vi "ESPECTROSCOPIA.vi"() -> ()   [LabVIEW 2016]
uses:
  Control 1.ctl
  <vilib>/userdefined/High Color/IMAQdx.ctl
  <vilib>/vision/driver/NI_Vision_Acquisition_Software.lvlib
panel:
  in  "worksheet index (0)":i32
  in  "entrada de datos desde un archivo":bool
  in  "Observar cámara":bool
  in  "Control de espejos":T1={"Movimiento de spot en y"=0.78, "Movimiento de spot en x"=0.5255, "tipo "=enum."barrido", "yFin"=0.82, "Paso"=0.01, "xFin"=0.5655} {"Movimiento de spot en x" scale=-10.0..10.0; "Movimiento de spot en y" min=-10.0 max=10.0 scale=-10.0..10.0}
  in  "arreglo opciones":bool[](array[boolean])=[FALSE, TRUE, TRUE, TRUE, FALSE]
  in  "Control CCD":T2={"Numero de lecturas"=0, "tiempo de lectura (ms)"=100, "Exposure"=0.053229, "Valor Gamma"=1.0, "Ganancia"=33, "Opción"=enum."Espectro", "VISA resource name"="", "Enable Strobe (Disabled)"=FALSE} {"Ganancia" min=0 max=100; "Valor Gamma" min=1.0 max=2.2; "Exposure" min=5e-05 max=0.053229}
  in  "Guardar":bool=TRUE
  in  "valor delay":u32=300
  in  "tiempo de avance":u32=300
  in  "Orden":T3(array[ring])=[enum."espejos", enum."voltaje", enum."polarizador", enum."CCD"]
  in  "Nombre del archivo":string="prueba280519PASO0.01_01_03"
  in  "stop medición":bool
  in  "stop":bool
  in  "Iniciar medición":bool
  in  "Config. fotodiodo y potenciometro":T4={"tiempo. lect."=300, "num. med"=20, "tiempo. lectura"=0, "average rate"=0, "Readout Config"="POW", "Tipo de Medición"=enum."Lockin", "usar multimetro"=FALSE}
  in  "config. Polarizador":T5={"pos inic"=0.0, "pos.final"=5.0, "incremento"=1.0, "velocidad"=0.0}
  in  "Config. voltaje y corriente":T6 {"Measurement Function (0:Voltage)" items=["Voltage", "Current", "Power"]; "Unit(V)" items=["V", "mV", "kV", "A", "mA"]; "Function(0:Voltage)" items=["Voltage", "Current"]}
  out "Imagen":T7(plugin-control)
  out "MULTÍMETRO":dbl format="%^#_9e"
  out "valor potenciometro":dbl format="%^#_9e"
  out "LockIn":dbl
  out "Valor voltaje":dbl
  out "corriente":dbl
  out "Ángulo del polarizador":dbl
  out "ysal":dbl=0.78
  out "xsal":dbl=0.5255
  out "division":T8
  out "multímetro":T8
  in  "Gráficas visibles":bool[](array[boolean])=[TRUE, FALSE, FALSE, FALSE, FALSE]
  in  "SerialNumber":string="55000538"
  out "I-V":cluster{dbl[], dbl[]}(graph)
  out "Gráfica general":T8
  out "Power meter":cluster{dbl[], dbl[]}(graph)
  # "Espejos"
  # "Polarizador"
  # "Fuente voltaje"
  # "Lockin \npotenciometro"
  # "CCD"
  # "Espectro"
  # "Imágen"
  # "Amplificador Lock in"
  # "potenciometro"
  # "Valores Numéricos"
  # "Gráfica general"
  # "Gráfica potenciómetro"
  # "Gráfica I-V"
  # "Multimetro"
  # "lockin/multimetro"
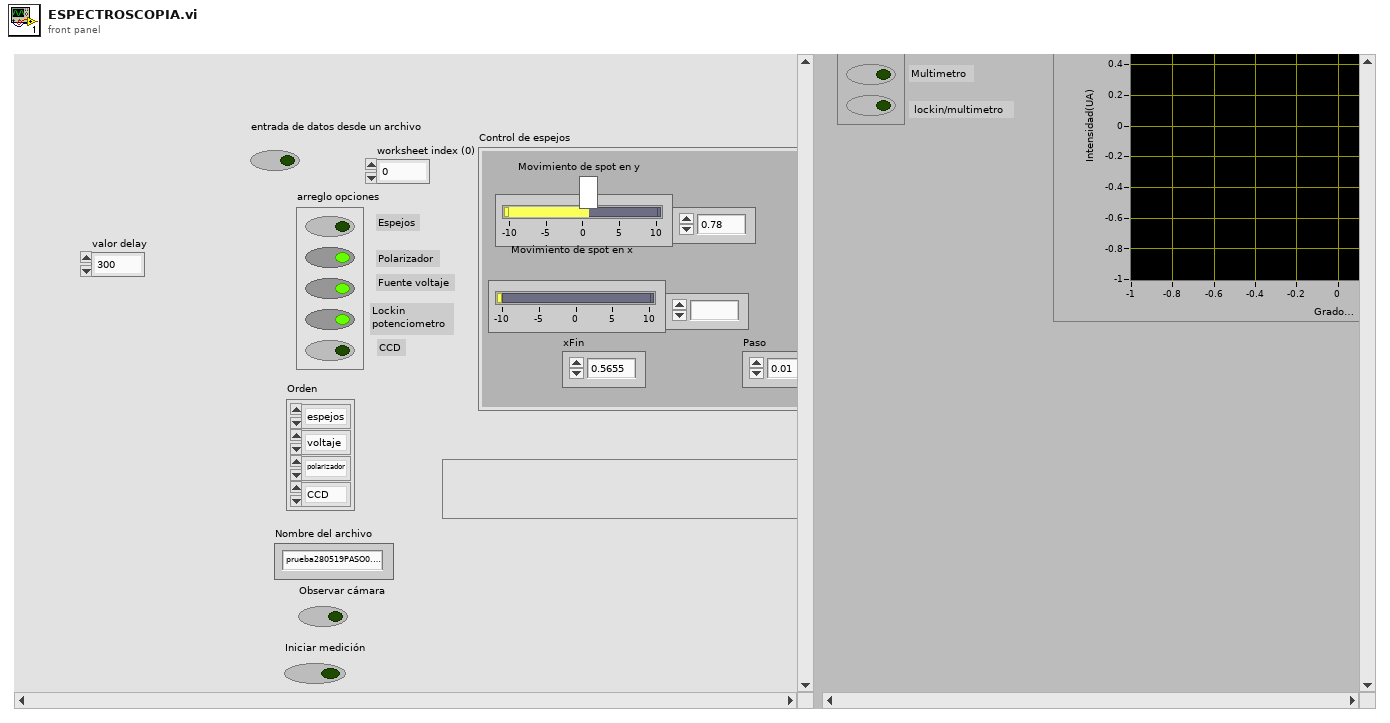
[diagram p1: front panel]
types:
  T1 = cluster{"Movimiento de spot en y":dbl, "Movimiento de spot en x":ext, "tipo ":enum16{"manual", "barrido"}, "yFin":dbl, "Paso":dbl, "xFin":dbl}
  T2 = cluster{"Numero de lecturas":i32, "tiempo de lectura (ms)":u32, "Exposure":dbl, "Valor Gamma":dbl, "Ganancia":i64, "Opción":enum16{"Espectro", "Imágen"}, "VISA resource name":refnum<visa-resource-name>, "Enable Strobe (Disabled)":bool}
  T3 = enum16{"espejos", "polarizador", "voltaje", "potenciometro y lockin", "CCD"}[]
  T4 = cluster{"tiempo. lect.":i32, "num. med":i32, "tiempo. lectura":i32, "average rate":i32, "Readout Config":string, "Tipo de Medición":enum16{"Lockin", "Lockin-potenciometro", "Potenciometro"}, "usar multimetro":bool}
  T5 = cluster{"pos inic":dbl, "pos.final":dbl, "incremento":dbl, "velocidad":dbl}
  T6 = cluster{"Voltaje inicial":dbl, "incremento":dbl, " voltaje final":dbl, "Function(0:Voltage)":u16, "Unit(V)":u16, "Measurement Function (0:Voltage)":u16, "VISA resource name":refnum<visa-resource-name>}
  T7 = typedef "IMAQ Image.ctl" = refnum<image>
  T8 = typedef "Control 1.ctl" = cluster{dbl[], dbl[]}
  T9 = typedef "IMAQdx.ctl" = refnum<k21>
  T10 = enum16{"espejos", "polarizador", "voltaje", "potenciometro y lockin", "CCD"}
  T11 = enum16{"Lockin", "Lockin-potenciometro", "Potenciometro"}
  T12 = cluster{"Global Rectangle":i32[], "Contours":cluster{"Contour Type":u32, "ROI Type":u32, "Points":i32[]}[]}
  T13 = cluster{"Wavelength (nm)":dbl[], "arreglo promedio":dbl[]}
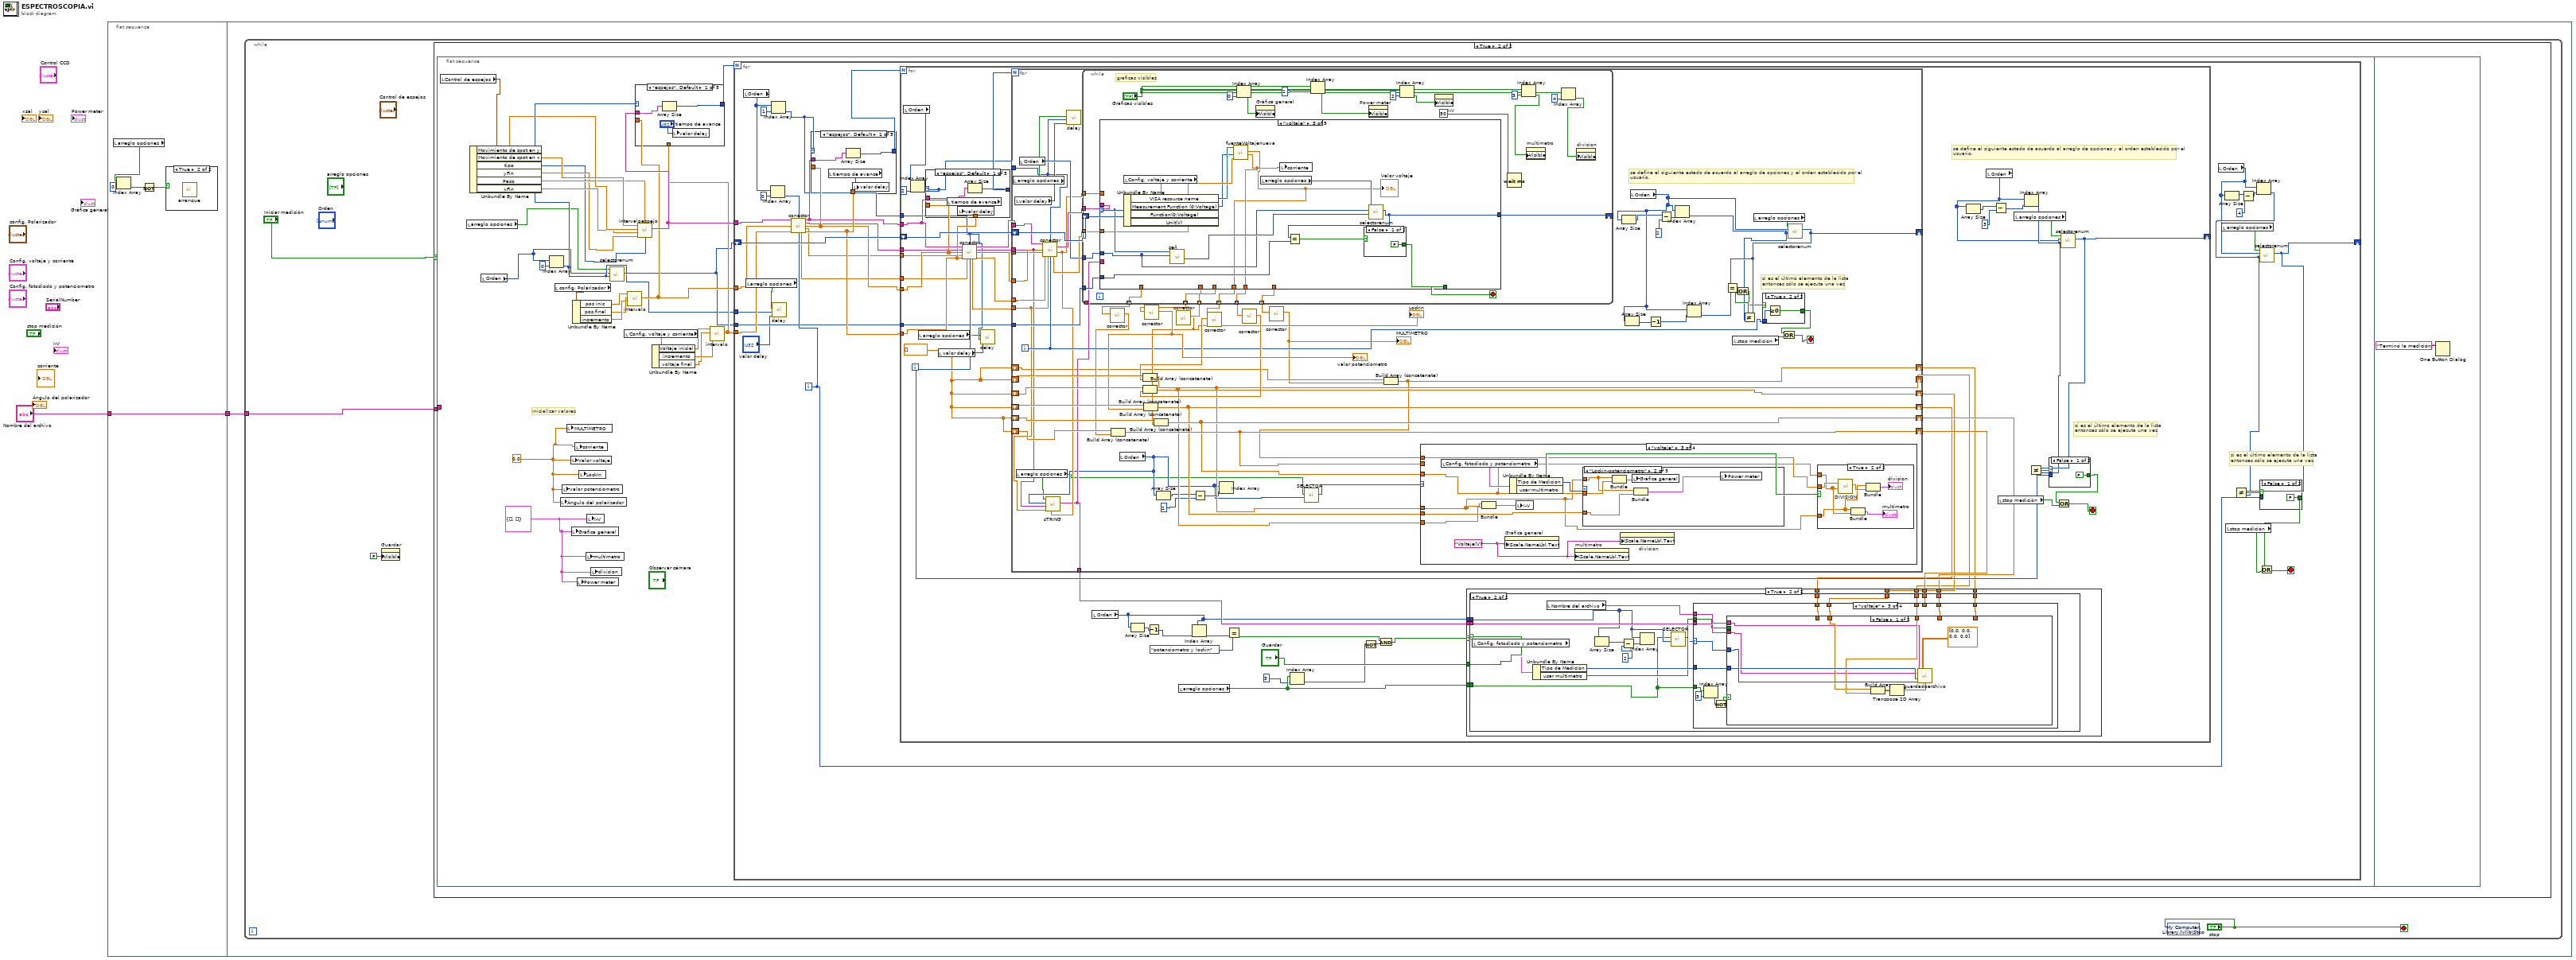
[diagram p0: block diagram]
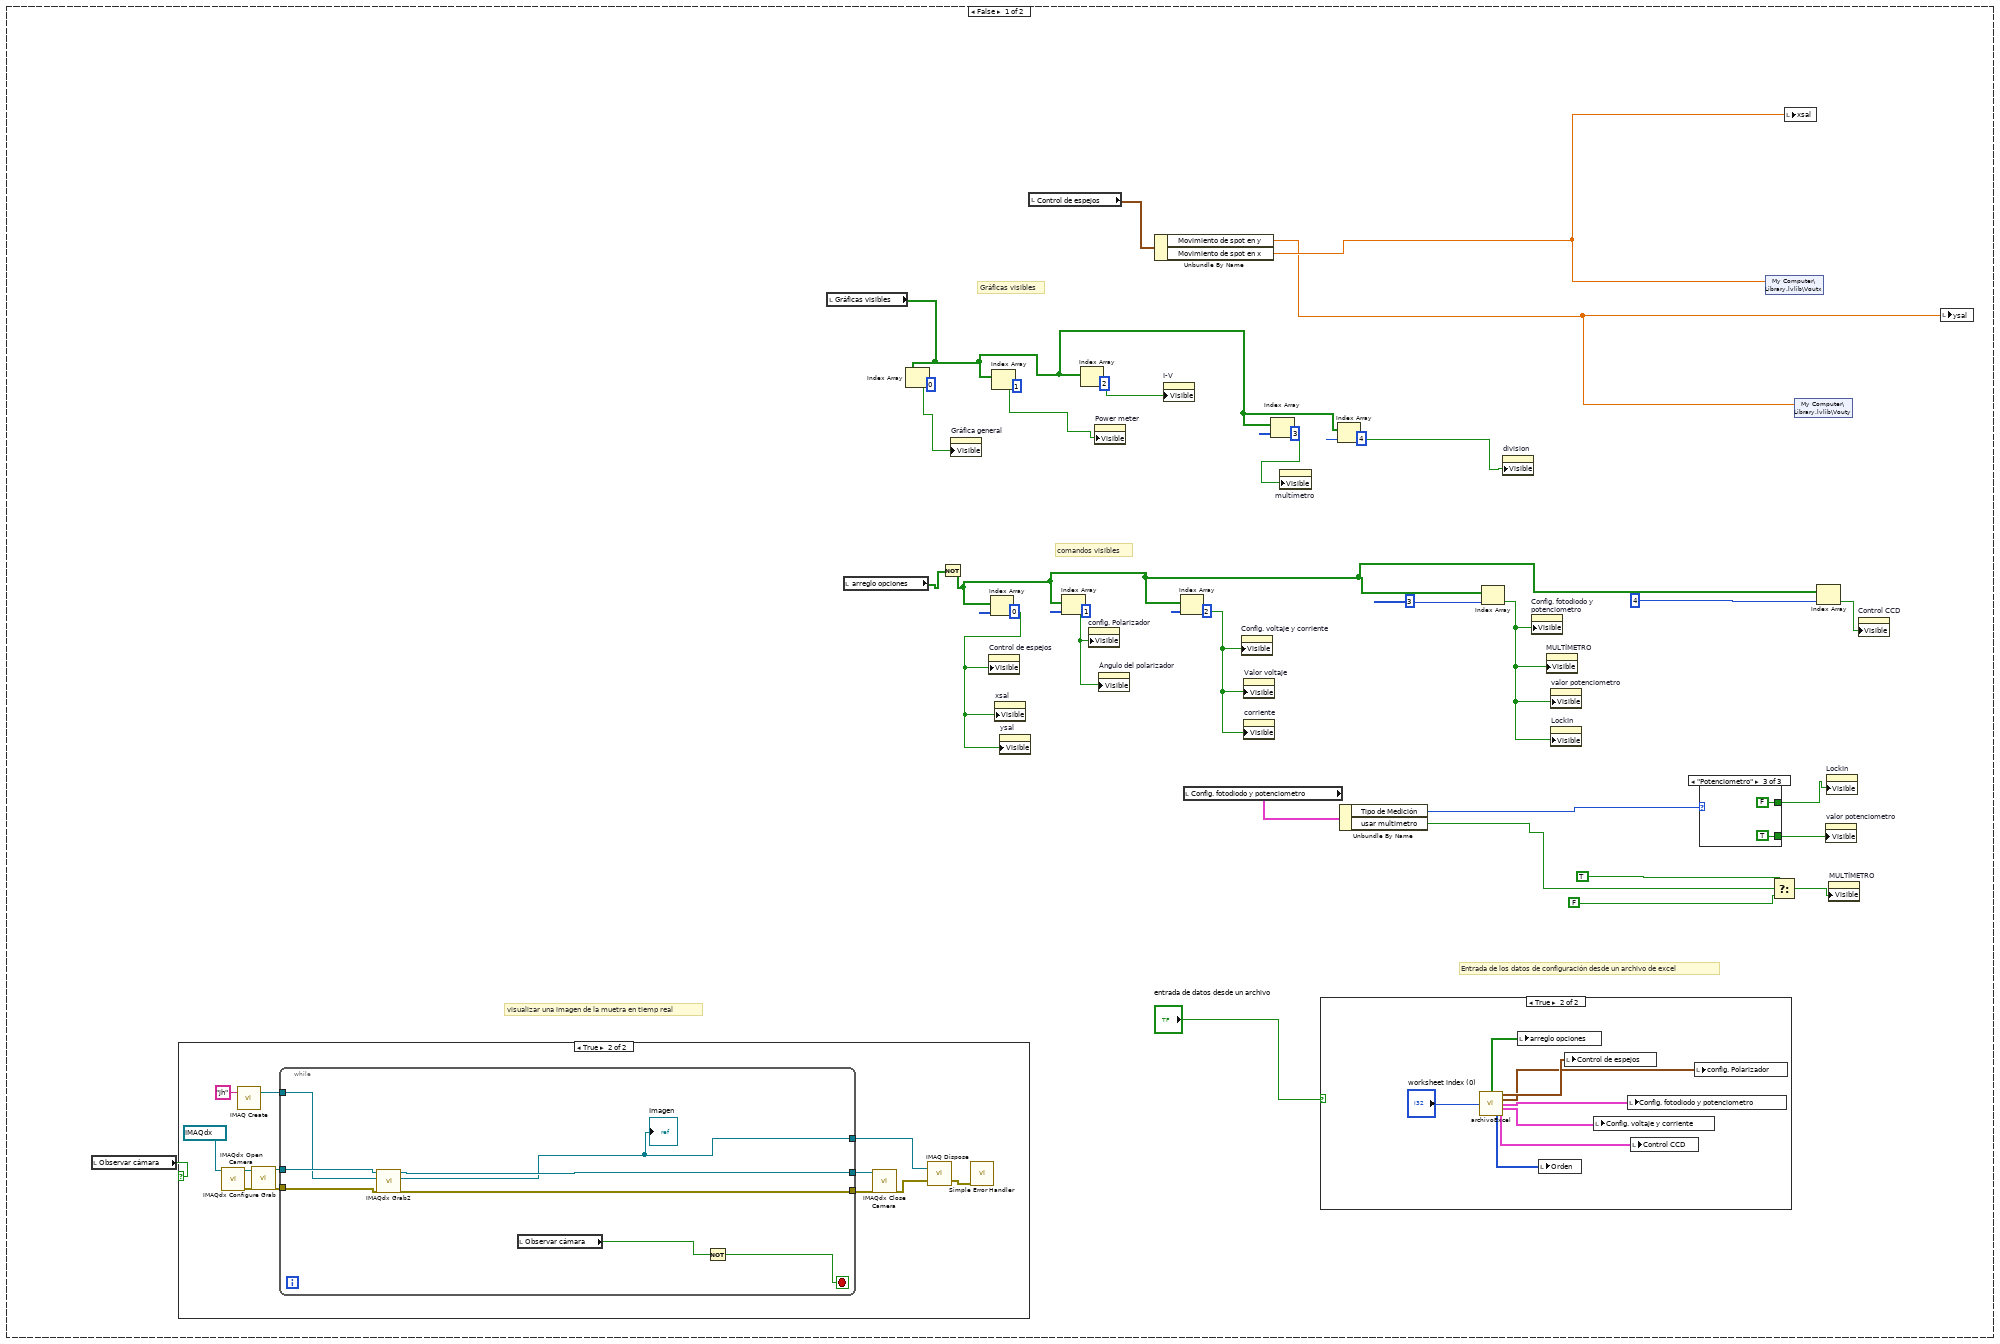
[diagram p3: hidden frame]
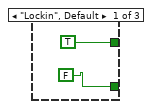
[diagram p6: hidden frame]
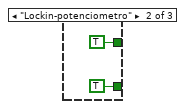
[diagram p7: hidden frame]
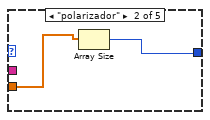
[diagram p8: hidden frame]
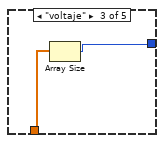
[diagram p9: hidden frame]
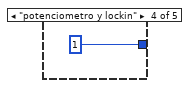
[diagram p10: hidden frame]
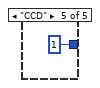
[diagram p11: hidden frame]
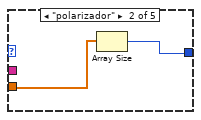
[diagram p12: hidden frame]
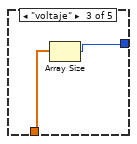
[diagram p13: hidden frame]
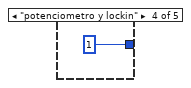
[diagram p14: hidden frame]
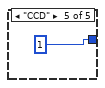
[diagram p15: hidden frame]
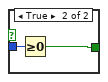
[diagram p16: hidden frame]
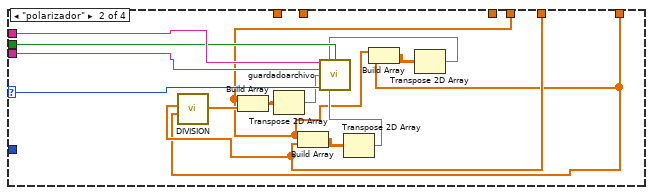
[diagram p20: hidden frame]
diagram:
  n1 = flat-sequence {
    tunnel: "Nombre del archivo" -> [w7]
    tunnel: [w7] -> w1
    tunnel: w1 -> [w8]
    frame #0 {
      n2 = local read "arreglo opciones"() -> (w6:bool[])
      n3 = Index Array(array=w6, index=0) -> (element=w3:bool)
      n4 = Not(x=w3) -> (.not. x?=w4:bool)
      n5 = case shown="True" w4 {
        frame False {
        }
        frame True {
          n6 = call "arranque.vi"() -> ()  [unwired: 12 in]
        }
      }
    }
    frame #1 {
      n7 = while {
        tunnel: w8 -> [w10]
        stop <- "stop" stop-if-true
        n8 = property on="Guardar" class="Bool (strict)"("Visible"=FALSE) -> ()  [unwired: 2 in, 2 out]
        n9 = case shown="True" "Iniciar medición" {
          tunnel: w10 -> [_ w83]
          frame False {
            # "Entrada de los datos de configuración desde un archivo de excel"
            # "visualizar una imagen de la muetra en tiemp real"
            # "comandos visibles"
            # "Gráficas visibles"
            n10 = local read "Observar cámara"() -> (w15:bool)
            n11 = case shown="True" w15 {
              frame False {
              }
              frame True {
                n12 = call <vilib>:"IMAQdx Open Camera.vi"("Session In"=T9 "cam4") -> ("error out"=w68:errorcluster, "Session Out"=w67:T9)  [unwired: 9 in]
                n13 = call "IMAQ Create"("Image Name"="jh") -> ("New Image"=w63:T7)  [unwired: 4 in, 1 out]
                n14 = call <vilib>:"IMAQdx Configure Grab.vi"("error in"=w68, "Session In"=w67) -> ("error out"=w65:errorcluster, "Session Out"=w66:T9)  [unwired: 8 in]
                n15 = while {
                  tunnel: w66 -> [w76]
                  tunnel: w65 -> [w75]
                  tunnel: w63 -> [w74]
                  tunnel: [w73] -> w61
                  tunnel: [w72] -> w60
                  tunnel: [w69] -> w58
                  stop <- w70 stop-if-true
                  n16 = call <vilib>:"IMAQdx Grab2.vi"("error in"=w75, "Image In"=w74, "Session In"=w76) -> ("error out"=w72:errorcluster, "Image Out"=w69:T7, "Session Out"=w73:T9)  [unwired: 5 in, 1 out]
                  "Imagen" <- w69
                  n17 = local read "Observar cámara"() -> (w71:bool)
                  n18 = Not(x=w71) -> (.not. x?=w70:bool)
                }
                n19 = call <vilib>:"IMAQdx Close Camera.vi"("error in"=w60, "Session In"=w61) -> ("error out"=w59:errorcluster)  [unwired: 9 in]
                n20 = call "IMAQ Dispose"("Image"=w58, "error in (no error)"=w59) -> ("error out"=w57:errorcluster)  [unwired: 4 in]
                n21 = call <vilib>:"Simple Error Handler.vi"("error in (no error)"=w57) -> ()  [unwired: 4 in, 5 out]
              }
            }
            n22 = local read "Gráficas visibles"() -> (w40:bool[])
            n23 = local read "arreglo opciones"() -> (w17:bool[])
            n24 = Index Array(array=w40, index=0) -> (element=w45:bool)
            n25 = Not(x=w17) -> (.not. x?=w16:bool[])
            n26 = property on="Gráfica general" class="XYGraph (strict)"("Visible"=w45) -> ()  [unwired: 2 in, 2 out]
            n27 = Index Array(array=w16, index=0) -> (element=w14:bool)
            n28 = property on="Control de espejos" class="Clust (strict)"("Visible"=w14) -> ()  [unwired: 2 in, 2 out]
            n29 = Index Array(array=w40, index=1) -> (element=w44:bool)
            n30 = property on="xsal" class="DigNum (strict)"("Visible"=w14) -> ()  [unwired: 2 in, 2 out]
            n31 = property on="ysal" class="DigNum (strict)"("Visible"=w14) -> ()  [unwired: 2 in, 2 out]
            n32 = local read "Control de espejos"() -> (w20:T1)
            n33 = Index Array(array=w16, index=1) -> (element=w35:bool)
            n34 = Index Array(array=w40, index=2) -> (element=w43:bool)
            n35 = property on="config. Polarizador" class="Clust (strict)"("Visible"=w35) -> ()  [unwired: 2 in, 2 out]
            n36 = property on="Power meter" class="XYGraph (strict)"("Visible"=w44) -> ()  [unwired: 2 in, 2 out]
            n37 = property on="Ángulo del polarizador" class="DigNum (strict)"("Visible"=w35) -> ()  [unwired: 2 in, 2 out]
            n38 = Unbundle By Name(w20) -> ("Movimiento de spot en y"=w18:dbl, "Movimiento de spot en x"=w19:ext)
            n39 = property on="I-V" class="XYGraph (strict)"("Visible"=w43) -> ()  [unwired: 2 in, 2 out]
            n40 = Index Array(array=w16, index=2) -> (element=w33:bool)
            n41 = local read "Config. fotodiodo y potenciometro"() -> (w28:T4)
            n42 = property on="Config. voltaje y corriente" class="Clust (strict)"("Visible"=w33) -> ()  [unwired: 2 in, 2 out]
            n43 = property on="Valor voltaje" class="DigNum (strict)"("Visible"=w33) -> ()  [unwired: 2 in, 2 out]
            n44 = property on="corriente" class="DigNum (strict)"("Visible"=w33) -> ()  [unwired: 2 in, 2 out]
            n45 = Index Array(array=w40, index=3) -> (element=w38:bool)
            n46 = property on="multímetro" class="XYGraph (strict)"("Visible"=w38) -> ()  [unwired: 2 in, 2 out]
            n47 = case shown="True" "entrada de datos desde un archivo" {
              frame False {
              }
              frame True {
                n48 = call "archivoExcel.vi"("worksheet index (0)"="worksheet index (0)") -> ("opciones"=w56:bool[], "Control de espejos 3"=w55:T1, "config. Polarizador 2"=w54:T5, "Config. fotodiodo y potenciometro 2"=w53:T4, "Config. voltaje y corriente 2"=w52:T6, "orden 2"=w50:T3, "Control CCD 2"=w51:T2)  [unwired: 8 in]
                n49 = local write "arreglo opciones"(w56) -> ()
                n50 = local write "Orden"(w50) -> ()
                n51 = local write "Control de espejos"(w55) -> ()
                n52 = local write "Config. voltaje y corriente"(w52) -> ()
                n53 = local write "Config. fotodiodo y potenciometro"(w53) -> ()
                n54 = local write "Control CCD"(w51) -> ()
                n55 = local write "config. Polarizador"(w54) -> ()
              }
            }
            n56 = Index Array(array=w40, index=4) -> (element=w39:bool)
            n57 = Unbundle By Name(w28) -> ("Tipo de Medición"=w27:T11, "usar multimetro"=w23:bool)
            n58 = Index Array(array=w16, index=3) -> (element=w31:bool)
            n59 = property on="division" class="XYGraph (strict)"("Visible"=w39) -> ()  [unwired: 2 in, 2 out]
            n60 = property on="Config. fotodiodo y potenciometro" class="Clust (strict)"("Visible"=w31) -> ()  [unwired: 2 in, 2 out]
            n61 = property on="MULTÍMETRO" class="DigNum (strict)"("Visible"=w31) -> ()  [unwired: 2 in, 2 out]
            n62 = property on="valor potenciometro" class="DigNum (strict)"("Visible"=w31) -> ()  [unwired: 2 in, 2 out]
            n63 = property on="LockIn" class="DigNum (strict)"("Visible"=w31) -> ()  [unwired: 2 in, 2 out]
            n64 = case shown="\"Potenciometro\"" w27 {
              tunnel: [TRUE TRUE FALSE] -> w26
              tunnel: [FALSE TRUE TRUE] -> w25
              frame "Lockin", Default {
              }
              frame "Lockin-potenciometro" {
              }
              frame "Potenciometro" {
              }
            }
            n65 = shared-variable "My Computer\\Library.lvlib\\Voutx"(w19) -> ()  [unwired: 1 in, 1 out]
            n66 = Select(t=TRUE, s=w23, f=FALSE) -> (s? t:f=w24:bool)
            n67 = local write "xsal"(w19) -> ()
            n68 = shared-variable "My Computer\\Library.lvlib\\Vouty"(w18) -> ()  [unwired: 1 in, 1 out]
            n69 = Index Array(array=w16, index=4) -> (element=w29:bool)
            n70 = property on="valor potenciometro" class="DigNum (strict)"("Visible"=w25) -> ()  [unwired: 2 in, 2 out]
            n71 = property on="LockIn" class="DigNum (strict)"("Visible"=w26) -> ()  [unwired: 2 in, 2 out]
            n72 = property on="MULTÍMETRO" class="DigNum (strict)"("Visible"=w24) -> ()  [unwired: 2 in, 2 out]
            n73 = property on="Control CCD" class="Clust (strict)"("Visible"=w29) -> ()  [unwired: 2 in, 2 out]
            n74 = local write "ysal"(w18) -> ()
          }
          frame True {
            n75 = flat-sequence {
              tunnel: w83 -> [_]
              frame #0 {
                w87 = cluster{dbl[], dbl[]} {[], []} ("I-V")
                w94 = 0.0
                # "Inicializar valores"
                n76 = local read "Control de espejos"() -> (w86:T1)
                n77 = local read "arreglo opciones"() -> (w85:bool[])
                n78 = Unbundle By Name(w86) -> ("Movimiento de spot en y"=w92:dbl, "Movimiento de spot en x"=w93:ext, "tipo"=w88:enum16{"manual", "barrido"}, "yFin"=w89:dbl, "Paso"=w91:dbl, "xFin"=w90:dbl)
                n79 = local read "Orden"() -> (w84:T3)
                n80 = Index Array(array=w84, index=0) -> (element=w95:T10)
                n81 = local read "config. Polarizador"() -> (w109:T5)
                n82 = local write "Ángulo del polarizador"(w94) -> ()
                n83 = local write "valor potenciometro"(w94) -> ()
                n84 = local write "MULTÍMETRO"(w94) -> ()
                n85 = local write "Valor voltaje"(w94) -> ()
                n86 = local write "Gráfica general"(w87) -> ()
                n87 = Unbundle By Name(w109) -> ("pos inic"=w108:dbl, "pos.final"=w106:dbl, "incremento"=w107:dbl)
                n88 = local write "corriente"(w94) -> ()
                n89 = local write "Power meter"(w87) -> ()
                n90 = local write "LockIn"(w94) -> ()
                n91 = local write "multímetro"(w87) -> ()
                n92 = local write "I-V"(w87) -> ()
                n93 = local write "division"(w87) -> ()
                n94 = call "selectorenum.vi"("Enum entrada"=w95, "Orden"=w84, "arreglo opciones"=w85) -> ("enum salida"=w96:T10)  [unwired: 8 in]
                n95 = local read "Config. voltaje y corriente"() -> (w105:T6)
                n96 = call "intervalo.vi"("incremento"=w107, "fin"=w106, "inicio"=w108) -> ("Array"=w98:dbl[])  [unwired: 8 in]
                n97 = call "intervaloespejo.vi"("tipo"=w88, "intervalo"=w91, "fin y"=w89, "fin x"=w90, "inicio y"=w92, "inicio x"=w93) -> ("salida"=w99:string[])  [unwired: 5 in]
                n98 = Unbundle By Name(w105) -> ("Voltaje inicial"=w104:dbl, "incremento"=w103:dbl, "voltaje final"=w102:dbl)
                n99 = call "intervalo.vi"("incremento"=w103, "fin"=w102, "inicio"=w104) -> ("Array"=w97:dbl[])  [unwired: 8 in]
                n100 = case shown="\"espejos\", Default" w95 {
                  tunnel: [w111 w113 w115 1 1] -> w100
                  tunnel: w99 -> [w112 _ _ _ _]
                  tunnel: w98 -> [_ w114 _ _ _]
                  tunnel: w97 -> [_ _ w116 _ _]
                  frame "espejos", Default {
                    n101 = Array Size(array=w112) -> (size(s)=w111:i32)
                    n102 = local write "valor delay"("tiempo de avance") -> ()
                  }
                  frame "polarizador" {
                    n103 = Array Size(array=w114) -> (size(s)=w113:i32)
                  }
                  frame "voltaje" {
                    n104 = Array Size(array=w116) -> (size(s)=w115:i32)
                  }
                  frame "potenciometro y lockin" {
                  }
                  frame "CCD" {
                  }
                }
                n105 = for {
                  N: w100 -> [_]
                  tunnel: w99 -> [w140]
                  shift-right: [w147] -> _
                  shift-left: w96 -> [w150]
                  tunnel: w98 -> [w139]
                  tunnel: w97 -> [w138]
                  tunnel: w96 -> [w130]
                  tunnel: w95 -> [w126]
                  i -> [w137]
                  stop <- w144 stop-if-true
                  # "si es el último elemento de la lista\nentonces sólo se ejecuta una vez"
                  n106 = local read "Orden"() -> (w129:T3)
                  n107 = local read "arreglo opciones"() -> (w125:bool[])
                  n108 = Index Array(array=w129, index=0) -> (element=w119:T10)
                  n109 = Index Array(array=w129, index=1) -> (element=w127:T10)
                  n110 = call "delay.vi"("valor delay"="valor delay", "element"=w126, "arreglo opciones"=w125) -> ()  [unwired: 9 in]
                  n111 = call "conector.vi"("salida"=w140, "Enum 2"=w119, "polarizador"=w139, "voltaje"=w138, "Indice"=w137) -> ("salida 2"=w136:string[], "Salida ent 2"=w133:string, "polarizador 2"=w135:dbl[], "Polarizador"=w132:dbl, "VoltajeEnt 2"=w131:dbl, "voltaje 2"=w134:dbl[])  [unwired: 5 in]
                  n112 = case shown="\"espejos\", Default" w127 {
                    tunnel: [w152 w154 w156 1 1] -> w143
                    tunnel: w136 -> [w153 _ _ _ _]
                    tunnel: w135 -> [_ w155 _ _ _]
                    tunnel: w134 -> [_ _ w157 _ _]
                    frame "espejos", Default {
                      n113 = local read "tiempo de avance"() -> (w151:u32)
                      n114 = Array Size(array=w153) -> (size(s)=w152:i32)
                      n115 = local write "valor delay"(w151) -> ()
                    }
                    frame "polarizador" {
                      n116 = Array Size(array=w155) -> (size(s)=w154:i32)
                    }
                    frame "voltaje" {
                      n117 = Array Size(array=w157) -> (size(s)=w156:i32)
                    }
                    frame "potenciometro y lockin" {
                    }
                    frame "CCD" {
                    }
                  }
                  n118 = for {
                    N: w143 -> [_]
                    tunnel: w136 -> [w201]
                    shift-right: [w213] -> _
                    shift-left: w150 -> [w215]
                    tunnel: w135 -> [w200]
                    tunnel: w134 -> [w199]
                    tunnel: w133 -> [w197]
                    tunnel: w132 -> [w196]
                    tunnel: w131 -> [w195]
                    tunnel: w130 -> [w194]
                    tunnel: w127 -> [w163]
                    i -> [w198]
                    stop <- w212 stop-if-true
                    w174 = dbl[] []
                    # "si es el último elemento de la lista\nentonces sólo se ejecuta una vez"
                    # "se define el siguiente estado de acuerdo al arreglo de opciones y el orden establecido por el \nusuario."
                    n119 = local read "Orden"() -> (w207:T3)
                    n120 = Index Array(array=w207, index=2) -> (element=w193:T10)
                    n121 = local read "arreglo opciones"() -> (w192:bool[])
                    n122 = case shown="\"espejos\", Default" w193 {
                      tunnel: [w302 w304 w306 1 1] -> w208
                      tunnel: w201 -> [w303 _ _ _ _]
                      tunnel: w200 -> [_ w305 _ _ _]
                      tunnel: w199 -> [_ _ w307 _ _]
                      frame "espejos", Default {
                        n123 = local read "tiempo de avance"() -> (w301:u32)
                        n124 = local write "valor delay"(w301) -> ()
                        n125 = Array Size(array=w303) -> (size(s)=w302:i32)
                      }
                      frame "polarizador" {
                        n126 = Array Size(array=w305) -> (size(s)=w304:i32)
                      }
                      frame "voltaje" {
                        n127 = Array Size(array=w307) -> (size(s)=w306:i32)
                      }
                      frame "potenciometro y lockin" {
                      }
                      frame "CCD" {
                      }
                    }
                    n128 = local read "valor delay"() -> (w191:u32)
                    n129 = call "conector.vi"("salida"=w201, "Enum 2"=w163, "Salida ent"=w197, "polarizador"=w200, "Polarizadorent"=w196, "voltaje"=w199, "VoltajeEnt"=w195, "Indice"=w198) -> ("salida 2"=w204:string[], "Salida ent 2"=w176:string, "polarizador 2"=w203:dbl[], "Polarizador"=w175:dbl, "VoltajeEnt 2"=w177:dbl, "voltaje 2"=w202:dbl[])  [unwired: 2 in]
                    n130 = call "delay.vi"("valor delay"=w191, "element"=w163, "arreglo opciones"=w192) -> ()  [unwired: 9 in]
                    n131 = for {
                      N: w208 -> [_]
                      shift-right: [w371] -> _
                      shift-left: w215 -> [w375]
                      tunnel: w204 -> [w352]
                      tunnel: w203 -> [w351]
                      tunnel: w202 -> [w350]
                      shift-right: [w338] -> w186
                      shift-left: w174 -> [w369]
                      shift-right: [w337] -> w187
                      shift-left: w174 -> [w368]
                      shift-right: [w336] -> w188
                      shift-left: w174 -> [w367]
                      shift-right: [w339] -> w189
                      shift-left: w174 -> [w366]
                      tunnel: w177 -> [w325]
                      tunnel: w175 -> [w346]
                      tunnel: w176 -> [w326]
                      tunnel: w194 -> [w344]
                      tunnel: w193 -> [w313]
                      shift-right: [w340] -> w190
                      shift-left: w174 -> [w342]
                      tunnel: [w322] -> w178
                      shift-right: [w319] -> w173
                      shift-left: w174 -> [w320]
                      i -> [w347]
                      stop <- w365 stop-if-true
                      # "si es el último elemento de la lista\nentonces sólo se ejecuta una vez"
                      # "se define el siguiente estado de acuerdo al arreglo de opciones y el orden establecido por el \nusuario."
                      n132 = local read "arreglo opciones"() -> (w334:bool[])
                      n133 = local read "valor delay"() -> (w333:u32)
                      n134 = local read "arreglo opciones"() -> (w314:bool[])
                      n135 = local read "Orden"() -> (w345:T3)
                      n136 = call "conector.vi"("salida"=w352, "Enum 2"=w313, "Salida ent"=w326, "polarizador"=w351, "Polarizadorent"=w346, "voltaje"=w350, "VoltajeEnt"=w325, "Indice"=w347) -> ("Salida ent 2"=w349:string, "Polarizador"=w324:dbl, "VoltajeEnt 2"=w348:dbl)  [unwired: 2 in, 3 out]
                      n137 = call "delay.vi"("valor delay"=w333, "element"=w313, "arreglo opciones"=w334) -> ()  [unwired: 9 in]
                      n138 = local read "Orden"() -> (w315:T3)
                      n139 = call "sTRING.vi"("angulo"=w324, "Valor del voltaje"=w325, "cadena entrada"=w326, "Orden"=w315, "arreglo opciones"=w314) -> ("String"=w322:string)  [unwired: 6 in]
                      n140 = while {
                        shift-right: [w444] -> _
                        shift-left: w375 -> [w445]
                        tunnel: w349 -> [w441]
                        tunnel: w324 -> [w442]
                        tunnel: w348 -> [w440]
                        tunnel: [w439] -> w359 mode=indexing
                        tunnel: [w438] -> w357 mode=indexing
                        tunnel: [w437] -> w360 mode=indexing
                        tunnel: [w436] -> w361 mode=indexing
                        tunnel: w345 -> [w434]
                        tunnel: w344 -> [w433]
                        tunnel: [w432] -> w343 mode=indexing
                        tunnel: w322 -> [w431]
                        tunnel: [w424] -> w321 mode=indexing
                        stop <- w443 stop-if-true
                        # "graficas visibles"
                        n141 = case shown="\"voltaje\"" w445 {
                          selector: w445 -> [w451 w462 w479 w492 w522]
                          tunnel: [w454 w466 w482 w504 w527] -> w444
                          tunnel: [w453 w468 w484 w505 w528] -> w443
                          tunnel: w442 -> [_ w465 _ _ _]
                          tunnel: w441 -> [w452 _ _ _ _]
                          tunnel: w440 -> [_ _ w474 _ _]
                          tunnel: [_ _ w475 _ _] -> w439
                          tunnel: [_ _ w476 _ _] -> w438
                          tunnel: [_ _ _ w502 _] -> w437
                          tunnel: [_ _ _ w501 _] -> w436
                          tunnel: w434 -> [w448 w461 w477 w490 w523]
                          tunnel: w433 -> [w449 w460 w480 w493 w526]
                          tunnel: [_ w459 _ _ _] -> w432
                          tunnel: w431 -> [_ _ _ _ w520]
                          tunnel: [_ _ _ w488 _] -> w424
                          frame "espejos", Default {
                            n142 = call "señ.vi"("Orden"=w448, "Enum"=w451) -> ("element"=w450:T10)  [unwired: 9 in]
                            n143 = call "controlespejo.vi"("cadena entrada"=w452) -> ("x"=w447:dbl, "y"=w446:dbl)  [unwired: 9 in]
                            n144 = local write "xsal"(w447) -> ()
                            n145 = local write "ysal"(w446) -> ()
                            n146 = local read "arreglo opciones"() -> (w456:bool[])
                            n147 = call "selectorenum.vi"("Enum entrada"=w450, "Orden"=w448, "arreglo opciones"=w456) -> ("enum salida"=w454:T10)  [unwired: 8 in]
                            n148 = Equal?(x=w454, y=w449) -> (x = y?=w455:bool)
                            n149 = case shown="True" w455 {
                              tunnel: [FALSE TRUE] -> w453
                              frame False {
                              }
                              frame True {
                              }
                            }
                          }
                          frame "polarizador" {
                            n150 = local read "SerialNumber"() -> (w464:string)
                            n151 = call "pol2.vi"("SerialNumber"=w464, "position"=w465) -> ("GetPositionCounter"=w459:dbl)  [unwired: 9 in]
                            n152 = call "señ.vi"("Orden"=w461, "Enum"=w462) -> ("element"=w463:T10)  [unwired: 9 in]
                            n153 = local write "Ángulo del polarizador"(w459) -> ()
                            n154 = local read "arreglo opciones"() -> (w469:bool[])
                            n155 = call "selectorenum.vi"("Enum entrada"=w463, "Orden"=w461, "arreglo opciones"=w469) -> ("enum salida"=w466:T10)  [unwired: 8 in]
                            n156 = Equal?(x=w466, y=w460) -> (x = y?=w467:bool)
                            n157 = case shown="True" w467 {
                              tunnel: [FALSE TRUE] -> w468
                              frame False {
                              }
                              frame True {
                              }
                            }
                          }
                          frame "voltaje" {
                            n158 = local read "Config. voltaje y corriente"() -> (w481:T6)
                            n159 = Unbundle By Name(w481) -> ("VISA resource name"=w473:refnum<visa-resource-name>, "Measurement Function (0:Voltage)"=w472:u16)  [unwired: 2 out]
                            n160 = call "señ.vi"("Orden"=w477, "Enum"=w479) -> ("element"=w478:T10)  [unwired: 9 in]
                            n161 = call "fuenteVoltajenueva.vi"("entrada"=w474, "Source Mode  (0: Voltage)"=w472, "VISA resource name"=w473) -> ("CORRIENTE"=w476:dbl, "VOLTAJE"=w475:dbl)  [unwired: 7 in]
                            "Valor voltaje" <- w475
                            n162 = local read "arreglo opciones"() -> (w485:bool[])
                            n163 = local write "corriente"(w476) -> ()
                            n164 = call "selectorenum.vi"("Enum entrada"=w478, "Orden"=w477, "arreglo opciones"=w485) -> ("enum salida"=w482:T10)  [unwired: 8 in]
                            n165 = Equal?(x=w482, y=w480) -> (x = y?=w483:bool)
                            n166 = case shown="False" w483 {
                              tunnel: [FALSE TRUE] -> w484
                              frame False {
                              }
                              frame True {
                              }
                            }
                          }
                          frame "potenciometro y lockin" {
                            n167 = local read "Config. fotodiodo y potenciometro"() -> (w500:T4)
                            n168 = Unbundle By Name(w500) -> ("tiempo. lect."=w499:i32, "num. med"=w494:i32, "tiempo. lectura"=w498:i32, "average rate"=w497:i32, "Readout Config"=w496:string, "Tipo de Medición"=w495:T11, "usar multimetro"=w489:bool)
                            n169 = call "controllockin.vi"("usar multimetro"=w489, "Enum"=w495, "num lecturas lockin"=w494, "Readout Config"=w496, "average rate"=w497, "tiempo lecturas potenciomtro"=w498, "tiempo lecturas lockin"=w499) -> ("multimetro"=w488:dbl, "valor potenciometro"=w501:dbl, "Valor Lockin"=w502:dbl)  [unwired: 2 in]
                            n170 = call "señ.vi"("Orden"=w490, "Enum"=w492) -> ("element"=w491:T10)  [unwired: 9 in]
                            n171 = local read "arreglo opciones"() -> (w506:bool[])
                            n172 = call "selectorenum.vi"("Enum entrada"=w491, "Orden"=w490, "arreglo opciones"=w506) -> ("enum salida"=w504:T10)  [unwired: 8 in]
                            n173 = Equal?(x=w493, y=w504) -> (x = y?=w503:bool)
                            n174 = case shown="True" w503 {
                              tunnel: [FALSE TRUE] -> w505
                              frame False {
                              }
                              frame True {
                              }
                            }
                          }
                          frame "CCD" {
                            n175 = local read "Control CCD"() -> (w509:T2)
                            n176 = property on="Imagen" class="ImageControl"() -> ("ROI"=w518:T12)  [unwired: 2 in, 2 out]
                            n177 = Unbundle By Name(w509) -> ("tiempo de lectura (ms)"=w510:u32, "Exposure"=w517:dbl, "Valor Gamma"=w516:dbl, "Ganancia"=w515:i64, "Opción"=w514:enum16{"Espectro", "Imágen"}, "VISA resource name"=w512:refnum<visa-resource-name>, "Enable Strobe (Disabled)"=w513:bool, "Numero de lecturas"=w511:i32)
                            n178 = Unbundle By Name(w518) -> ("Global Rectangle"=w519:i32[])
                            n179 = local read "Nombre del archivo"() -> (w521:string)
                            n180 = case shown="\"Imágen\"" w514 {
                              tunnel: w521 -> [w536 w551]
                              tunnel: w520 -> [w535 w550]
                              tunnel: w510 -> [_ w548]
                              tunnel: w519 -> [_ w547]
                              tunnel: w517 -> [_ w546]
                              tunnel: w516 -> [_ w545]
                              tunnel: w515 -> [_ w544]
                              tunnel: w513 -> [w543 _]
                              tunnel: w512 -> [w542 _]
                              tunnel: w511 -> [w541 _]
                              tunnel: w510 -> [w540 _]
                              frame "Espectro", Default {
                                n181 = call "espectroCCD.vi"("Enable Strobe (Disabled)"=w543, "tiempo de lectura (ms)"=w540, "Numero de lecturas"=w541, "VISA resource name"=w542) -> ("arreglo promedio"=w532:dbl[], "Wavelength (nm)"=w533:dbl[])  [unwired: 6 in]
                                n182 = Build Array(w533, w532) -> (w531:dbl[][])
                                n183 = Bundle("Wavelength (nm)"=w533, "arreglo promedio"=w532) -> (w539:T13)  [unwired: 1 in]
                                n184 = Transpose 2D Array(2D array=w531) -> (transposed array=w530:dbl[][])
                                n185 = property on="Gráfica general" class="XYGraph (strict)"("XScale.NameLbl.Text"="Lamda(nm)" ("X Scale.Name Label.Text")) -> ()  [unwired: 2 in, 2 out]
                                n186 = property on="Gráfica general" class="XYGraph (strict)"("YScale.NameLbl.Text"="Reflectancia(UA)" ("Y Scale.Name Label.Text")) -> ()  [unwired: 2 in, 2 out]
                                n187 = local write "Gráfica general"(w539) -> ()
                                n188 = call "guardadoarchivo.vi"("nombre"=w536, "CCD"=w530, "titulo grupo"=w535, "element"=T10."CCD") -> ()  [unwired: 12 in]
                              }
                              frame "Imágen" {
                                n189 = call "imagenCam.vi"("Valor Gamma"=w545, "Ganancia"=w544, "Exposure"=w546, "tiempo de exposición (ms)"=w548, "titulo grupo"=w550, "nombre"=w551, "Optional Rectangle"=w547) -> ("Image"=w549:T7)  [unwired: 3 in, 1 out]
                                n190 = local write "Imagen"(w549) -> ()
                              }
                            }
                            n191 = call "señ.vi"("Orden"=w523, "Enum"=w522) -> ("element"=w525:T10)  [unwired: 9 in]
                            n192 = local read "arreglo opciones"() -> (w524:bool[])
                            n193 = call "selectorenum.vi"("Enum entrada"=w525, "Orden"=w523, "arreglo opciones"=w524) -> ("enum salida"=w527:T10)  [unwired: 8 in]
                            n194 = Equal?(x=w527, y=w526) -> (x = y?=w529:bool)
                            n195 = case shown="True" w529 {
                              tunnel: [FALSE TRUE] -> w528
                              frame False {
                              }
                              frame True {
                              }
                            }
                          }
                        }
                        n196 = Index Array(array="Gráficas visibles", index=0) -> (element=w429:bool)
                        n197 = property on="Gráfica general" class="XYGraph (strict)"("Visible"=w429) -> ()  [unwired: 2 in, 2 out]
                        n198 = Index Array(array="Gráficas visibles", index=1) -> (element=w425:bool)
                        n199 = property on="Power meter" class="XYGraph (strict)"("Visible"=w425) -> ()  [unwired: 2 in, 2 out]
                        n200 = Index Array(array="Gráficas visibles", index=2) -> (element=w430:bool)
                        n201 = property on="I-V" class="XYGraph (strict)"("Visible"=w430) -> ()  [unwired: 2 in, 2 out]
                        n202 = Wait (ms)(milliseconds to wait=u32 50) -> ()  [unwired: 1 out]
                        n203 = Index Array(array="Gráficas visibles", index=3) -> (element=w420:bool)
                        n204 = property on="multímetro" class="XYGraph (strict)"("Visible"=w420) -> ()  [unwired: 2 in, 2 out]
                        n205 = Index Array(array="Gráficas visibles", index=4) -> (element=w419:bool)
                        n206 = property on="division" class="XYGraph (strict)"("Visible"=w419) -> ()  [unwired: 2 in, 2 out]
                      }
                      n207 = call "corrector.vi"("Array"=w343) -> ("valor salida"=w341:dbl)  [unwired: 10 in]
                      n208 = Build Array (concatenate)(w342, w341) -> (w340:dbl[])
                      n209 = call "corrector.vi"("Array"=w361) -> ("valor salida"=w362:dbl)  [unwired: 10 in]
                      "valor potenciometro" <- w362
                      n210 = Build Array (concatenate)(w367, w362) -> (w336:dbl[])
                      n211 = Array Size(array=w315) -> (size(s)=w331:i32)
                      n212 = call "corrector.vi"("Array"=w360) -> ("valor salida"=w355:dbl)  [unwired: 10 in]
                      "LockIn" <- w355
                      n213 = Build Array (concatenate)(w366, w355) -> (w339:dbl[])
                      n214 = Subtract(x=w331, y=2 ("index")) -> (x-y=w332:i32)
                      n215 = call "corrector.vi"("Array"=w359) -> ("valor salida"=w358:dbl)  [unwired: 10 in]
                      n216 = Build Array (concatenate)(w369, w358) -> (w338:dbl[])
                      n217 = Index Array(array=w315, index=w332) -> ()  [unwired: 1 out]
                      n218 = call "corrector.vi"("Array"=w357) -> ("valor salida"=w356:dbl)  [unwired: 10 in]
                      n219 = Build Array (concatenate)(w368, w356) -> (w337:dbl[])
                      n220 = call "corrector.vi"("Array"=w321) -> ("valor salida"=w317:dbl)  [unwired: 10 in]
                      "MULTÍMETRO" <- w317
                      n221 = call "SELECTOR.vi"("Orden"=w315, "arreglo opciones"=w314) -> ("Enum"=w316:T10)  [unwired: 9 in]
                      n222 = Build Array (concatenate)(w320, w317) -> (w319:dbl[])
                      n223 = case shown="\"voltaje\"" w316 {
                        tunnel: w340 -> [_ w381 _ _]
                        tunnel: w339 -> [_ w376 w390 _]
                        tunnel: w338 -> [_ _ w391 _]
                        tunnel: w337 -> [_ _ w395 _]
                        tunnel: w336 -> [_ _ w394 _]
                        tunnel: w319 -> [_ w377 w392 _]
                        frame "espejos", Default {
                        }
                        frame "polarizador" {
                          w378 = "Grados(°)" ("Y Scale.Name Label.Text")
                          n224 = local read "Config. fotodiodo y potenciometro"() -> (w379:T4)
                          n225 = Bundle(w381, w376) -> (w382:cluster{dbl[], dbl[]})  [unwired: 1 in]
                          n226 = local write "Gráfica general"(w382) -> ()
                          n227 = property on="multímetro" class="XYGraph (strict)"("XScale.NameLbl.Text"=w378) -> ()  [unwired: 2 in, 2 out]
                          n228 = property on="Gráfica general" class="XYGraph (strict)"("XScale.NameLbl.Text"=w378) -> ()  [unwired: 2 in, 2 out]
                          n229 = Unbundle By Name(w379) -> ("usar multimetro"=w380:bool)
                          n230 = case shown="True" w380 {
                            tunnel: w376 -> [_ w388]
                            tunnel: w381 -> [_ w385]
                            tunnel: w377 -> [_ w387]
                            frame False {
                            }
                            frame True {
                              n231 = call "DIVISION.vi"("r"=w387, "dr"=w388) -> ("dr/r"=w386:dbl[])  [unwired: 9 in]
                              n232 = Bundle(w385, w387) -> (w383:cluster{dbl[], dbl[]})  [unwired: 1 in]
                              n233 = Bundle(w385, "dr/r"=w386) -> (w384:cluster{dbl[], "dr/r":dbl[]})  [unwired: 1 in]
                              n234 = local write "multímetro"(w383) -> ()
                              n235 = local write "division"(w384) -> ()
                            }
                          }
                          n236 = property on="division" class="XYGraph (strict)"("XScale.NameLbl.Text"=w378) -> ()  [unwired: 2 in, 2 out]
                        }
                        frame "voltaje" {
                          w389 = "Voltaje(V)" ("Y Scale.Name Label.Text")
                          n237 = local read "Config. fotodiodo y potenciometro"() -> (w398:T4)
                          n238 = Bundle(w391, w395) -> (w396:cluster{dbl[], dbl[]})  [unwired: 1 in]
                          n239 = property on="Gráfica general" class="XYGraph (strict)"("XScale.NameLbl.Text"=w389) -> ()  [unwired: 2 in, 2 out]
                          n240 = Unbundle By Name(w398) -> ("Tipo de Medición"=w397:T11, "usar multimetro"=w393:bool)
                          n241 = local write "I-V"(w396) -> ()
                          n242 = property on="multímetro" class="XYGraph (strict)"("XScale.NameLbl.Text"=w389) -> ()  [unwired: 2 in, 2 out]
                          n243 = case shown="\"Lockin-potenciometro\"" w397 {
                            tunnel: w391 -> [w407 w410 w414]
                            tunnel: w390 -> [w406 w411 _]
                            tunnel: w394 -> [_ w409 w413]
                            frame "Lockin", Default {
                              n244 = Bundle(w407, w406) -> (w405:cluster{dbl[], dbl[]})  [unwired: 1 in]
                              n245 = local write "Gráfica general"(w405) -> ()
                            }
                            frame "Lockin-potenciometro" {
                              n246 = Bundle(w410, w411) -> (w412:cluster{dbl[], dbl[]})  [unwired: 1 in]
                              n247 = local write "Gráfica general"(w412) -> ()
                              n248 = Bundle(w410, w409) -> (w408:cluster{dbl[], dbl[]})  [unwired: 1 in]
                              n249 = local write "Power meter"(w408) -> ()
                            }
                            frame "Potenciometro" {
                              n250 = Bundle(w414, w413) -> (w415:cluster{dbl[], dbl[]})  [unwired: 1 in]
                              n251 = local write "Power meter"(w415) -> ()
                            }
                          }
                          n252 = property on="division" class="XYGraph (strict)"("XScale.NameLbl.Text"=w389) -> ()  [unwired: 2 in, 2 out]
                          n253 = case shown="True" w393 {
                            tunnel: w392 -> [_ w403]
                            tunnel: w391 -> [_ w400]
                            tunnel: w390 -> [_ w402]
                            frame False {
                            }
                            frame True {
                              n254 = call "DIVISION.vi"("r"=w402, "dr"=w403) -> ("dr/r"=w401:dbl[])  [unwired: 9 in]
                              n255 = Bundle(w400, w402) -> (→"multímetro":cluster{dbl[], dbl[]})  [unwired: 1 in]
                              n256 = Bundle(w400, "dr/r"=w401) -> (→"division":cluster{dbl[], "dr/r":dbl[]})  [unwired: 1 in]
                            }
                          }
                        }
                        frame "potenciometro y lockin" {
                        }
                      }
                      n257 = local read "Orden"() -> (w318:T3)
                      n258 = Array Size(array=w318) -> (size(s)=w328:i32)
                      n259 = Array Size(array=w318) -> (size(s)=w354:i32)
                      n260 = Decrement(x=w354) -> (x-1=w353:i32)
                      n261 = Subtract(x=w328, y=2 ("index")) -> (x-y=w329:i32)
                      n262 = Index Array(array=w318, index=w329) -> (element=w335:T10)
                      n263 = Index Array(array=w318, index=w353) -> (element=w323:T10)
                      n264 = local read "stop medición"() -> (w363:bool)
                      n265 = local read "arreglo opciones"() -> (w374:bool[])
                      n266 = call "selectorenum.vi"("Enum entrada"=w335, "Orden"=w318, "arreglo opciones"=w374) -> ("enum salida"=w371:T10)  [unwired: 8 in]
                      n267 = Equal?(x=w371, y=w323) -> (x = y?=w372:bool)
                      n268 = Not Equal?(x=w371, y=w335) -> (x != y?=w373:bool)
                      n269 = Or(x=w372, y=w373) -> (x .or. y?=w370:bool)
                      n270 = case shown="True" w370 {
                        tunnel: [FALSE w418] -> w364
                        tunnel: w347 -> [_ w417]
                        frame False {
                        }
                        frame True {
                          n271 = Greater Or Equal To 0?(x=w417) -> (x >= 0?=w418:bool)
                        }
                      }
                      n272 = Or(x=w364, y=w363) -> (x .or. y?=w365:bool)
                    }
                    n273 = local read "Orden"() -> (w166:T3)
                    n274 = Array Size(array=w166) -> (size(s)=w165:i32)
                    n275 = Decrement(x=w165) -> (x-1=w164:i32)
                    n276 = local read "arreglo opciones"() -> (w170:bool[])
                    n277 = Index Array(array=w166, index=w164) -> (element=w180:T10)
                    n278 = Equal?(x=T10."potenciometro y lockin", y=w180) -> (x = y?=w172:bool)
                    n279 = Index Array(array=w170, index=3) -> (element=w167:bool)
                    n280 = Not(x=w167) -> (.not. x?=w168:bool)
                    n281 = And(x=w172, y=w168) -> (x .and. y?=w171:bool)
                    n282 = case shown="True" w171 {
                      tunnel: w190 -> [_ w225]
                      tunnel: w189 -> [_ w224]
                      tunnel: w178 -> [_ w223]
                      tunnel: w188 -> [_ w222]
                      tunnel: w187 -> [_ w221]
                      tunnel: w186 -> [_ w220]
                      tunnel: "Guardar" -> [_ w219]
                      tunnel: w166 -> [_ w218]
                      tunnel: w173 -> [_ w217]
                      tunnel: w170 -> [_ w216]
                      frame False {
                      }
                      frame True {
                        n283 = case shown="True" w219 {
                          tunnel: w225 -> [_ w242]
                          tunnel: w224 -> [_ w241]
                          tunnel: w223 -> [_ w240]
                          tunnel: w222 -> [_ w236]
                          tunnel: w221 -> [_ w235]
                          tunnel: w220 -> [_ w234]
                          tunnel: w218 -> [_ w228]
                          tunnel: w217 -> [_ w229]
                          tunnel: w216 -> [_ w226]
                          frame False {
                          }
                          frame True {
                            n284 = local read "Config. fotodiodo y potenciometro"() -> (w238:T4)
                            n285 = Unbundle By Name(w238) -> ("Tipo de Medición"=w237:T11, "usar multimetro"=w230:bool)
                            n286 = local read "Nombre del archivo"() -> (w239:string)
                            n287 = Array Size(array=w228) -> (size(s)=w231:i32)
                            n288 = Subtract(x=w231, y=2 ("index")) -> (x-y=w232:i32)
                            n289 = Index Array(array=w228, index=w232) -> ()  [unwired: 1 out]
                            n290 = call "SELECTOR.vi"("Orden"=w228, "arreglo opciones"=w226) -> ("Enum"=w227:T10)  [unwired: 9 in]
                            n291 = case shown="\"voltaje\"" w227 {
                              selector: w227 -> [_ w252 w268 _]
                              tunnel: w242 -> [_ w244 _ _]
                              tunnel: w241 -> [_ w247 w264 _]
                              tunnel: w240 -> [_ w254 w269 _]
                              tunnel: w239 -> [_ w255 w270 _]
                              tunnel: w237 -> [_ _ w267 _]
                              tunnel: w236 -> [_ _ w266 _]
                              tunnel: w235 -> [_ _ w265 _]
                              tunnel: w234 -> [_ _ w263 _]
                              tunnel: w230 -> [_ w251 w261 _]
                              tunnel: w229 -> [_ w243 w262 _]
                              tunnel: w226 -> [_ _ w260 _]
                              frame "espejos", Default {
                              }
                              frame "polarizador" {
                                n292 = call "DIVISION.vi"("r"=w243, "dr"=w247) -> ("dr/r"=w248:dbl[])  [unwired: 9 in]
                                n293 = Build Array(w244, w248) -> (w250:dbl[][])
                                n294 = Transpose 2D Array(2D array=w250) -> (transposed array=w249:dbl[][])
                                n295 = Build Array(w244, w247) -> (w256:dbl[][])
                                n296 = Transpose 2D Array(2D array=w256) -> (transposed array=w253:dbl[][])
                                n297 = Build Array(w244, w243) -> (w246:dbl[][])
                                n298 = Transpose 2D Array(2D array=w246) -> (transposed array=w245:dbl[][])
                                n299 = call "guardadoarchivo.vi"("nombre"=w255, "lockin"=w245, "multimetro"=w251, "titulo grupo"=w254, "potenciometro"=w249, "element"=w252, "polarizador"=w253) -> ()  [unwired: 9 in]
                              }
                              frame "voltaje" {
                                n300 = Index Array(array=w260, index=3) -> (element=w258:bool)
                                n301 = Not(x=w258) -> (.not. x?=w257:bool)
                                n302 = case shown="False" w257 {
                                tunnel: w270 -> [w273 w300]
                                tunnel: w269 -> [w272 w299]
                                tunnel: w268 -> [w279 w298]
                                tunnel: w267 -> [w278 w297]
                                tunnel: w266 -> [_ w292]
                                tunnel: w265 -> [w277 w286]
                                tunnel: w264 -> [_ w285]
                                tunnel: w263 -> [w276 w283]
                                tunnel: w262 -> [_ w282]
                                tunnel: w261 -> [_ w280]
                                frame False {
                                n303 = Build Array(w277, w276) -> (w275:dbl[][])
                                n304 = Transpose 2D Array(2D array=w275) -> (transposed array=w274:dbl[][])
                                n305 = call "guardadoarchivo.vi"("nombre"=w273, "lockin"=dbl[][] [[0.0, 0.0], [0.0, 0.0]], "titulo grupo"=w272, "Tipo de Medición"=w278, "element"=w279, "corriente"=w274) -> ()  [unwired: 10 in]
                                }
                                frame True {
                                n306 = Build Array(w283, w292) -> (w294:dbl[][])
                                n307 = Transpose 2D Array(2D array=w294) -> (transposed array=w293:dbl[][])
                                n308 = call "DIVISION.vi"("r"=w282, "dr"=w285) -> ("dr/r"=w287:dbl[])  [unwired: 9 in]
                                n309 = Build Array(w283, w286) -> (w296:dbl[][])
                                n310 = Build Array(w283, w287) -> (w288:dbl[][])
                                n311 = Build Array(w283, w282) -> (w284:dbl[][])
                                n312 = Transpose 2D Array(2D array=w296) -> (transposed array=w295:dbl[][])
                                n313 = Transpose 2D Array(2D array=w288) -> (transposed array=w289:dbl[][])
                                n314 = Transpose 2D Array(2D array=w284) -> (transposed array=w281:dbl[][])
                                n315 = Build Array(w283, w285) -> (w290:dbl[][])
                                n316 = Transpose 2D Array(2D array=w290) -> (transposed array=w291:dbl[][])
                                n317 = call "guardadoarchivo.vi"("nombre"=w300, "lockin"=w291, "multimetro"=w280, "titulo grupo"=w299, "potenciometro"=w293, "Tipo de Medición"=w297, "element"=w298, "polarizador"=w289, "corriente"=w295, "multim."=w281) -> ()  [unwired: 6 in]
                                }
                                }
                              }
                              frame "potenciometro y lockin" {
                              }
                            }
                          }
                        }
                      }
                    }
                    n318 = local read "Orden"() -> (w185:T3)
                    n319 = Array Size(array=w185) -> (size(s)=w184:i32)
                    n320 = Subtract(x=w184, y=3 ("index")) -> (x-y=w182:i32)
                    n321 = local read "stop medición"() -> (w210:bool)
                    n322 = local read "arreglo opciones"() -> (w209:bool[])
                    n323 = Index Array(array=w185, index=w182) -> (element=w205:T10)
                    n324 = call "selectorenum.vi"("Enum entrada"=w205, "Orden"=w185, "arreglo opciones"=w209) -> ("enum salida"=w213:T10)  [unwired: 8 in]
                    n325 = Not Equal?(x=w213, y=w205) -> (x != y?=w214:bool)
                    n326 = case shown="False" w214 {
                      tunnel: [FALSE w311] -> w211
                      tunnel: w198 -> [_ w312]
                      frame False {
                      }
                      frame True {
                        n327 = Greater Or Equal To 0?(x=w312) -> (x >= 0?=w311:bool)
                      }
                    }
                    n328 = Or(x=w211, y=w210) -> (x .or. y?=w212:bool)
                  }
                  n329 = local read "Orden"() -> (w124:T3)
                  n330 = local read "arreglo opciones"() -> (w148:bool[])
                  n331 = Array Size(array=w124) -> (size(s)=w122:i32)
                  n332 = local read "stop medición"() -> (w146:bool)
                  n333 = Subtract(x=w122, y=4 ("index")) -> (x-y=w123:i32)
                  n334 = Index Array(array=w124, index=w123) -> (element=w141:T10)
                  n335 = call "selectorenum.vi"("Enum entrada"=w141, "Orden"=w124, "arreglo opciones"=w148) -> ("enum salida"=w147:T10)  [unwired: 8 in]
                  n336 = Not Equal?(x=w147, y=w141) -> (x != y?=w149:bool)
                  n337 = case shown="False" w149 {
                    tunnel: [FALSE w162] -> w145
                    tunnel: w137 -> [_ w161]
                    frame False {
                    }
                    frame True {
                      n338 = Greater Or Equal To 0?(x=w161) -> (x >= 0?=w162:bool)
                    }
                  }
                  n339 = Or(x=w145, y=w146) -> (x .or. y?=w144:bool)
                }
              }
              frame #1 {
                n340 = One Button Dialog(message="Terminó la medición.") -> ()  [unwired: 1 in, 1 out]
              }
            }
          }
        }
        n341 = shared-variable "My Computer\\Library.lvlib\\Stop"("stop") -> ()  [unwired: 1 in, 1 out]
      }
    }
  }
